vi "MDPtr PointerTotalCount.vi"(8 "error in (no error)":errorcluster) -> (0 "error out":errorcluster, 2 "MDPtr Total Count":i64)   [LabVIEW 2014]
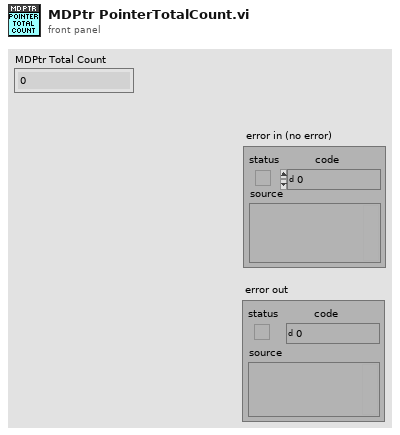
[diagram p1: front panel]
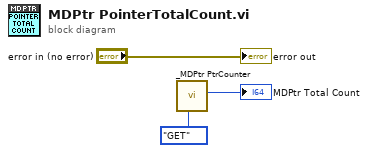
[diagram p0: block diagram]
diagram:
  n1 = call "_MDPtr PtrCounter.vi"("Oper(Get)"=enum16{"GET", "Increament", "decreament"}."GET") -> ("Value out"=→"MDPtr Total Count":i64)  [unwired: 9 in, 1 out]
  "error out" <- "error in (no error)"
